vi "read_current_vision_tuning.vi"(10 "OpenCV to LV":dbl, 11 "Current Filter in":T1) -> (3 "Current Filter out":T1)   [LabVIEW 2020]
uses:
  <vilib>/Rock Robotics/Network Tables/NT Read Number.vi
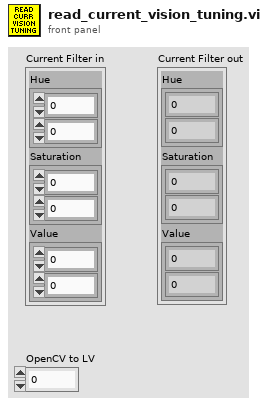
[diagram p1: front panel]
types:
  T1 = cluster{"Hue":cluster{dbl, dbl}, "Saturation":cluster{dbl, dbl}, "Value":cluster{dbl, dbl}}
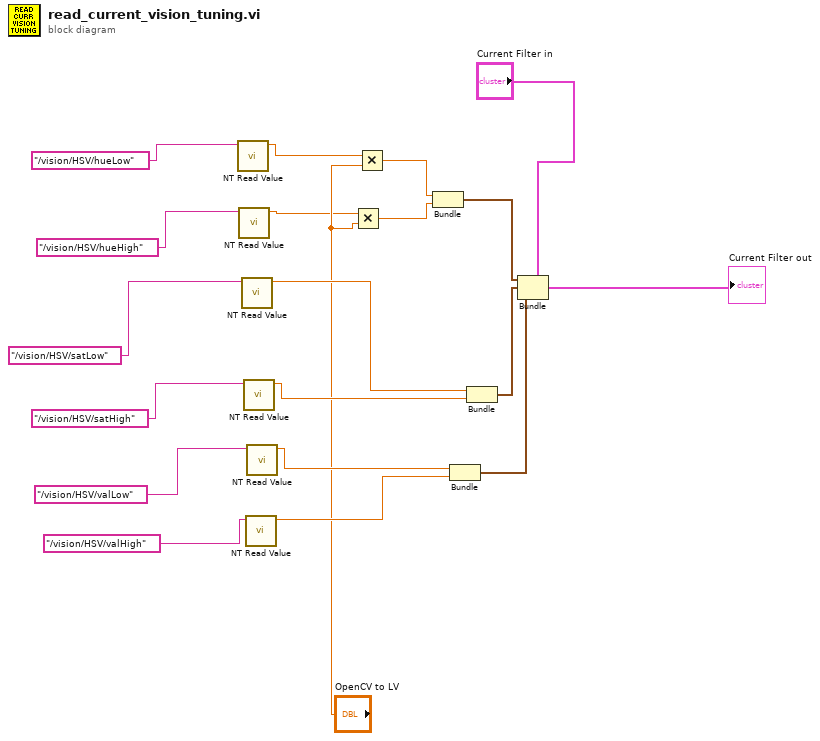
[diagram p0: block diagram]
diagram:
  n1 = call-poly <vilib>:"NT Read Value.vi"("name"="/vision/HSV/hueLow") -> ("value"=w7:dbl)  [unwired: 8 in, 2 out]
  n2 = call-poly <vilib>:"NT Read Value.vi"("name"="/vision/HSV/hueHigh") -> ("value"=w8:dbl)  [unwired: 8 in, 2 out]
  n3 = call-poly <vilib>:"NT Read Value.vi"("name"="/vision/HSV/satLow") -> ("value"=w12:dbl)  [unwired: 8 in, 2 out]
  n4 = call-poly <vilib>:"NT Read Value.vi"("name"="/vision/HSV/satHigh") -> ("value"=w13:dbl)  [unwired: 8 in, 2 out]
  n5 = call-poly <vilib>:"NT Read Value.vi"("name"="/vision/HSV/valHigh") -> ("value"=w15:dbl)  [unwired: 8 in, 2 out]
  n6 = call-poly <vilib>:"NT Read Value.vi"("name"="/vision/HSV/valLow") -> ("value"=w14:dbl)  [unwired: 8 in, 2 out]
  n7 = Multiply(x=w8, y="OpenCV to LV") -> (x*y=w11:dbl)
  n8 = Multiply(x=w7, y="OpenCV to LV") -> (x*y=w10:dbl)
  n9 = Bundle(w10, w11) -> (w16:cluster{dbl, dbl})  [unwired: 1 in]
  n10 = Bundle("value"=w14, "value"=w15) -> (w18:cluster{"value":dbl, "value":dbl})  [unwired: 1 in]
  n11 = Bundle("value"=w12, "value"=w13) -> (w17:cluster{"value":dbl, "value":dbl})  [unwired: 1 in]
  n12 = Bundle(cluster="Current Filter in", "Hue"=w16, "Saturation"=w17, "Value"=w18) -> (→"Current Filter out":T1)
